vi "ClassNode_CastToMoreSpecific.vi"(0 "reference":T1, 5 "error in (no error)":errorcluster) -> (14 "reference out":T1, 15 "Exists?":bool, 16 "IsSubclass?":bool, 19 "error out":errorcluster)   [LabVIEW 2016, in "ClassNode.lvclass"]
doc: "Casts object to SubSubClass."
uses:
  <resource>/Framework/Providers/Open_GDS/UML/ClassNode_class/ClassNode.lvclass
  <vilib>/addons/_goop2.llb/GOOPStates.ctl
  <resource>/Framework/Providers/Open_GDS/UML/AbstractNode_class/ObjectReference.ctl
  <resource>/Framework/Providers/Open_GDS/UML/AbstractNode_class/AbstractNode.lvclass
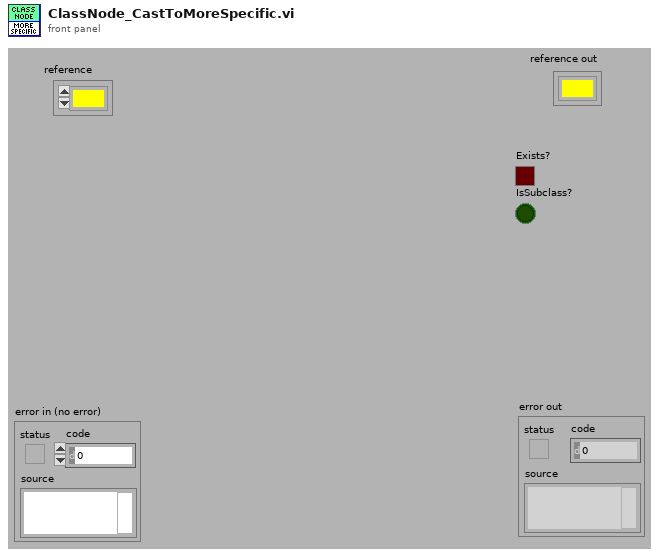
[diagram p1: front panel]
types:
  T1 = typedef "AbstractNode.lvclass/ObjectReference.ctl" = refnum<k1>
  T2 = typedef "GOOPStates.ctl" = enum16{"Set", "Get", "New", "Delete", "Clear", "Test and get", "Unlock data", "Information", "Look up existing", "New or look up existing", "Test and get shared", "Get shared", "Set shared", "Unlock shared", "Find dynamic method", "Register dynamic method", "Preload dynamic method", "Probe", "Cast to more generic", "Cast to more specific"}
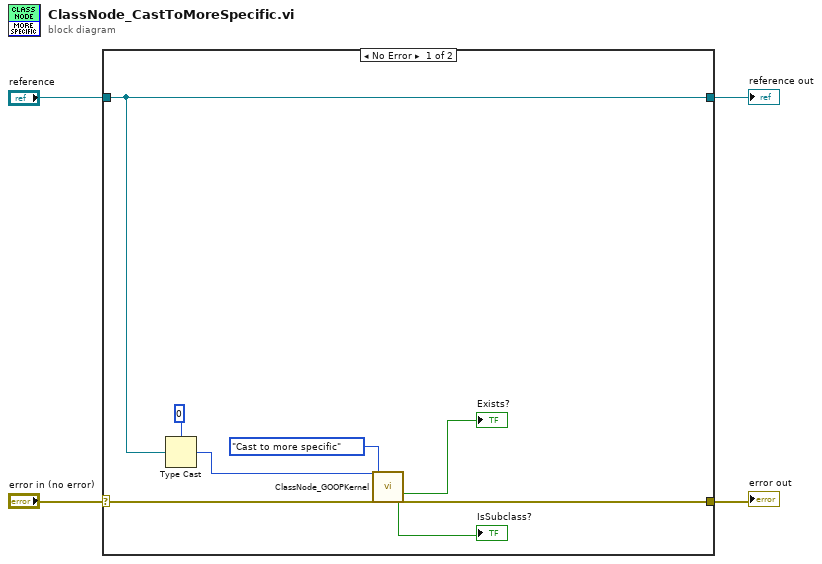
[diagram p0: block diagram]
diagram:
  n1 = case shown="No Error" "error in (no error)" {
    selector: "error in (no error)" -> [w12 w14]
    tunnel: [w11 w14] -> w3
    tunnel: "reference" -> [w9 w13]
    tunnel: [w9 w13] -> w2
    frame No Error {
      n2 = Type Cast(type=0, x=w9) -> (*(type *) &x=w7:i32)
      n3 = call <resource>:"ClassNode_GOOPKernel.vi"("Ref in"=w7, "error in (no error)"=w12, "Action"=GOOPStates."Cast to more specific") -> ("IsSubclass?"=→"IsSubclass?":bool, "Exists?"=→"Exists?":bool, "error out"=w11:errorcluster)  [unwired: 12 in, 10 out]
    }
    frame Error {
    }
  }
  "error out" <- w3
  "reference out" <- w2
